vi "例程41-基于逐点VI的滤波.vi"() -> ()   [LabVIEW 2016]
uses:
  <vilib>/Analysis/3filter.llb/Butterworth Filter (DBL).vi
  <vilib>/ptbypt/NI_PtbyPt.lvlib
  <vilib>/Analysis/NI_AALBase.lvlib
panel:
  in  "停止":bool
  out "基于数组滤波的信号":dbl[](graph)
  out "逐点滤波信号":dbl(graph)
  out "原始信号":dbl(graph)
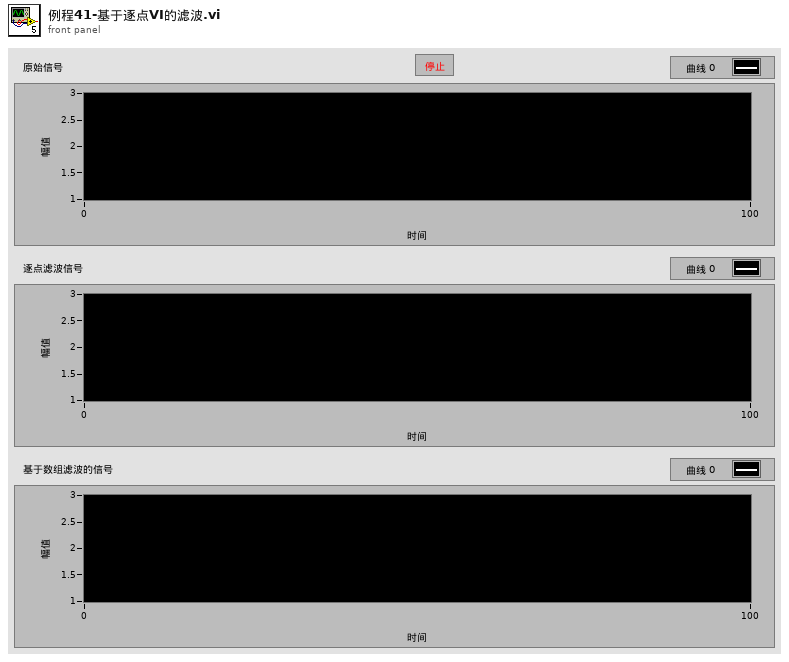
[diagram p1: front panel]
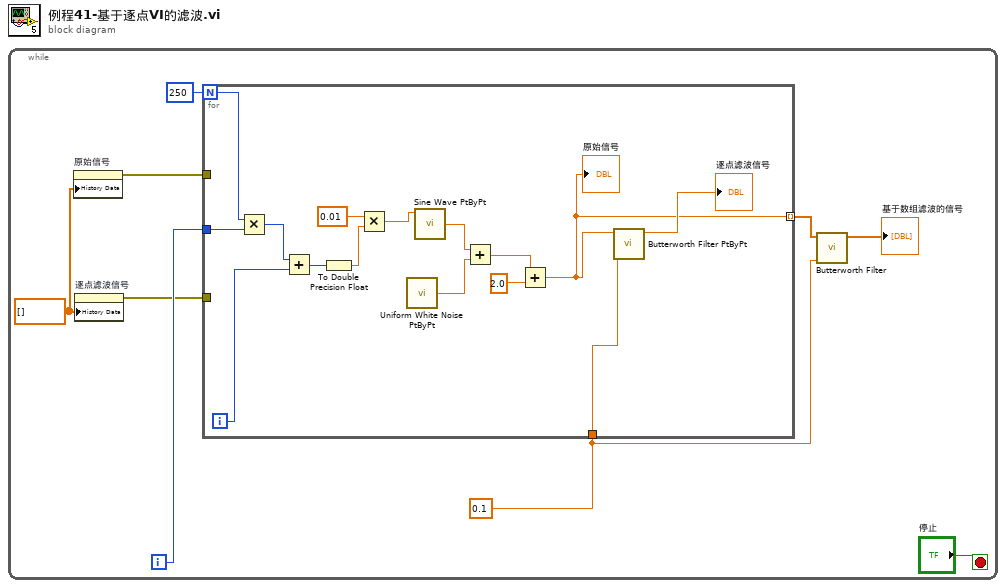
[diagram p0: block diagram]
diagram:
  n1 = while {
    i -> [w8]
    stop <- "停止" stop-if-true
    w1 = dbl[] [] ("历史数据")
    w6 = 0.1 ("low cutoff freq: fl")
    n2 = property on="原始信号" class="WFChart (严格)"("History Data"=w1) -> (error out=w3:errorcluster)  [unwired: 2 in, 1 out]
    n3 = property on="逐点滤波信号" class="WFChart (严格)"("History Data"=w1) -> (error out=w2:errorcluster)  [unwired: 2 in, 1 out]
    n4 = for {
      N: 250 -> [w12]
      tunnel: w6 -> [w19]
      tunnel: w8 -> [w11]
      tunnel: [w10] -> w7 mode=indexing
      tunnel: w3 -> [_]
      tunnel: w2 -> [_]
      i -> [w14]
      n5 = Multiply(x=w12, y=w11) -> (x*y=w13:i32)
      n6 = Add(x=w13, y=w14) -> (x+y=w17:i32)
      n7 = To Double Precision Float(number=w17) -> (double precision float=w16:dbl)
      n8 = Multiply(x=0.01, y=w16) -> (x*y=w24:dbl)
      n9 = call <vilib>:"Uniform White Noise PtByPt.vi"() -> ("uniform white noise"=w22:dbl)  [unwired: 3 in]
      n10 = call <vilib>:"Sine Wave PtByPt.vi"("amplitude"=w24) -> ("sine wave"=w23:dbl)  [unwired: 3 in]
      n11 = Add(x=w23, y=w22) -> (x+y=w21:dbl)
      n12 = Add(x=w21, y=2.0) -> (x+y=w10:dbl)
      "原始信号" <- w10
      n13 = call <vilib>:"Butterworth Filter PtByPt.vi"("low cutoff freq: fl"=w19, "x"=w10) -> ("Filtered x"=→"逐点滤波信号":dbl)  [unwired: 7 in, 1 out]
    }
    n14 = call-poly <vilib>:"Butterworth Filter.vi"("low cutoff freq: fl"=w6, "X"=w7) -> ("Filtered X"=→"基于数组滤波的信号":dbl[])  [unwired: 6 in, 1 out]
  }
